vi "calculateGraphData.vi"(7 "Online Buffer (1000)":i32=1000, 8 "error in":errorcluster, 9 "Offset in":i64, 10 "DataBuffers in":dbl[][](array[numeric]), 11 "GraphData in":cluster{dbl[], dbl[]}[](array[cluster])) -> (0 "error out":errorcluster, 3 "GraphData out":cluster{dbl[], dbl[]}[](array[cluster]))   [LabVIEW 2022 SP3, in "StreamReader.lvlib"]
uses:
  <instrlib>/openDAQ/Examples/StreamReader/StreamReader.lvlib
  <vilib>/Utility/miscctls.llb/LVDateTimeRec.ctl
  <vilib>/regexp/Match Regular Expression.xnode
  <instrlib>/openDAQ/Public/Classes/daqUtils/daqUtils.lvlib
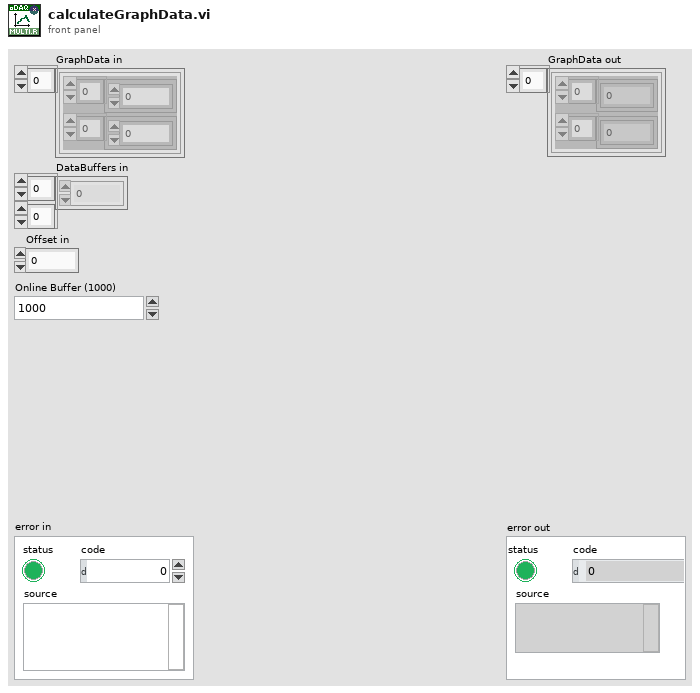
[diagram p1: front panel]
types:
  T1 = enum16{"init", "read", "set sampleRate", "set ruleStart", "set ruleDelta", "set referenceDomainOffset", "set origin", "set unitSymbol", "set resNum", "set resDen", " calculate sampleRate"}
  T2 = typedef "LVDateTimeRec.ctl" = cluster{"fractional second":dbl, "second":i32, "minute":i32, "hour":i32, "day of month":i32, "month":i32, "year":i32, "day of week":i32, "day of year":i32, "DST":i32}
  T3 = typedef "openDAQ.lvlib/DomainMetadata.ctl" = cluster{"sampleRate":i64, "ruleStart":i64, "ruleDelta":i64, "referenceDomainOffset":i64, "origin":string, "unitSymbol":string, "resNum":i64, "resDen":i64}
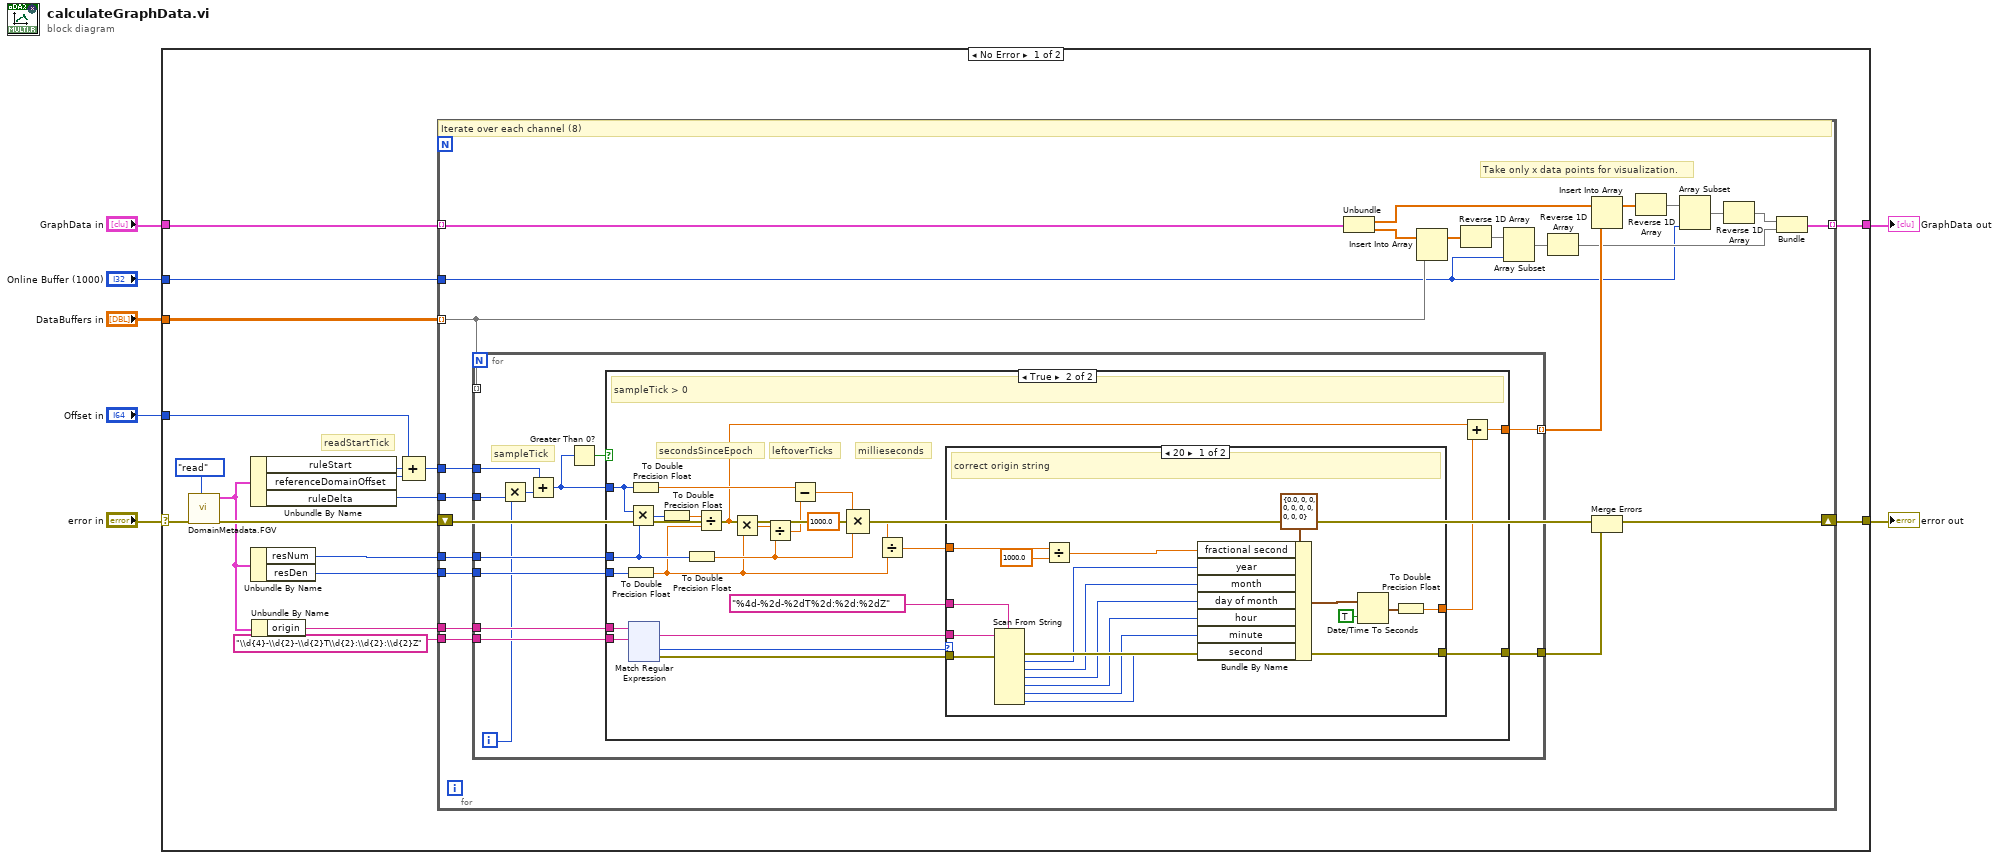
[diagram p0: block diagram]
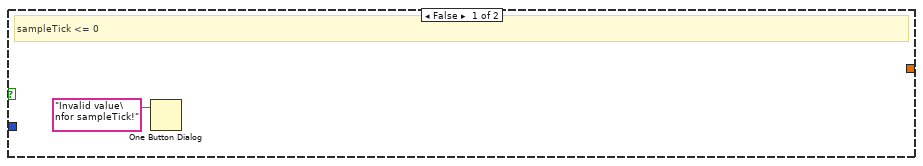
[diagram p2: hidden frame]
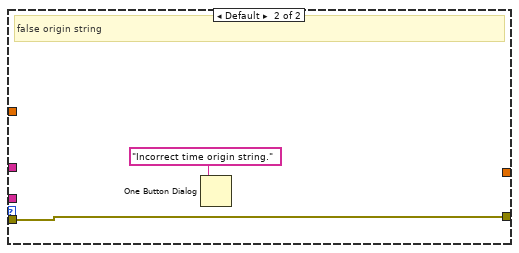
[diagram p3: hidden frame]
diagram:
  n1 = case shown="No Error" "error in" {
    selector: "error in" -> [w9 w225]
    tunnel: [w21 w225] -> w7
    tunnel: "DataBuffers in" -> [w13 _]
    tunnel: "Offset in" -> [w12 _]
    tunnel: "GraphData in" -> [w11 w224]
    tunnel: [w10 w224] -> w3
    tunnel: "Online Buffer (1000)" -> [w8 _]
    frame No Error {
      # "readStartTick"
      n2 = call <instrlib>:"DomainMetadata.FGV.vi"("Case Select"=T1."read", "error in"=w9) -> ("error out"=w22:errorcluster, "DomainMetadata out"=w16:T3)  [unwired: 8 in]
      n3 = Unbundle By Name(w16) -> ("ruleStart"=w24:i64, "referenceDomainOffset"=w23:i64, "ruleDelta"=w19:i64)
      n4 = Unbundle By Name(w16) -> ("resNum"=w18:i64, "resDen"=w17:i64)
      n5 = Unbundle By Name(w16) -> ("origin"=w15:string)
      n6 = Compound Arithmetic op=ADD(w12, w24, w23) -> (w20:i64)
      n7 = for {
        shift-right: [w41] -> w21
        shift-left: w22 -> [w45]
        tunnel: w20 -> [w48]
        tunnel: w19 -> [w49]
        tunnel: w18 -> [w47]
        tunnel: w17 -> [w46]
        tunnel: w15 -> [w44]
        tunnel: "\\d{4}-\\d{2}-\\d{2}T\\d{2}:\\d{2}:\\d{2}Z" ("format string") -> [w43]
        tunnel: w13 -> [w27] mode=indexing
        tunnel: [w39] -> w10 mode=indexing
        tunnel: w11 -> [w38] mode=indexing
        tunnel: w8 -> [w26]
        # "Take only x data points for visualization."
        # "Iterate over each channel (8)"
        n8 = for {
          tunnel: w49 -> [w61]
          tunnel: w48 -> [w59]
          tunnel: w47 -> [w57]
          tunnel: w46 -> [w56]
          tunnel: w44 -> [w54]
          tunnel: w43 -> [w53]
          tunnel: [w52] -> w42
          tunnel: w27 -> [_] mode=indexing
          tunnel: [w50] -> w40 mode=indexing
          i -> [w51]
          # "sampleTick"
          n9 = Multiply(x=w51, y=w61) -> (x*y=w60:i64)
          n10 = Add(x=w59, y=w60) -> (x+y=w55:i64)
          n11 = Greater Than 0?(x=w55) -> (x > 0?=w58:bool)
          n12 = case shown="True" w58 {
            tunnel: w57 -> [_ w82]
            tunnel: w56 -> [_ w84]
            tunnel: w55 -> [_ w81]
            tunnel: w54 -> [_ w69]
            tunnel: w53 -> [_ w73]
            tunnel: [_ w70] -> w52
            tunnel: [_ w63] -> w50
            frame False {
              # "sampleTick <= 0"
              n13 = One Button Dialog(message="Invalid value\nfor sampleTick!") -> ()  [unwired: 1 in, 1 out]
            }
            frame True {
              # "millieseconds"
              # "leftoverTicks"
              # "secondsSinceEpoch"
              # "sampleTick > 0"
              n14 = To Double Precision Float(number=w84) -> (double precision float=w74:dbl)
              n15 = Multiply(x=w81, y=w82) -> (x*y=w86:i64)
              n16 = xnode "Match Regular Expression"("input string"=w69, "regular expression"=w73) -> ("whole match"=w71:string, "offset past match"=w68:i32, "error out"=w67:errorcluster)  [unwired: 4 in, 2 out]
              n17 = To Double Precision Float(number=w81) -> (double precision float=w79:dbl)
              n18 = To Double Precision Float(number=w86) -> (double precision float=w85:dbl)
              n19 = To Double Precision Float(number=w82) -> (double precision float=w76:dbl)
              n20 = Divide(x=w85, y=w74) -> (x/y=w65:dbl)
              n21 = Multiply(x=w65, y=w74) -> (x*y=w83:dbl)
              n22 = Divide(x=w83, y=w76) -> (x/y=w80:dbl)
              n23 = Subtract(x=w79, y=w80) -> (x-y=w78:dbl)
              n24 = Compound Arithmetic op=MULTIPLY(w78, 1000.0 ("x/y"), w76) -> (w75:dbl)
              n25 = Divide(x=w75, y=w74) -> (x/y=w66:dbl)
              n26 = case shown="20" w68 {
                tunnel: "%4d-%2d-%2dT%2d:%2d:%2dZ" ("format string") -> [w220 _]
                tunnel: w71 -> [w219 _]
                tunnel: [w221 w222] -> w70
                tunnel: w67 -> [w218 w222]
                tunnel: [w208 _] -> w64
                tunnel: w66 -> [w206 _]
                frame 20 {
                  # "correct origin string"
                  n27 = Scan From String(format string=w220, input string=w219, error in=w218) -> (error out=w221:errorcluster, output 1=w216:i32, output 2=w215:i32, output 3=w214:i32, output 4=w213:i32, output 5=w212:i32, output 6=w211:i32)  [unwired: 7 in, 2 out]
                  n28 = Divide(x=w206, y=1000.0) -> (x/y=w204:dbl)
                  n29 = Bundle By Name(cluster=T2 {"fractional second"=0.0, "second"=0, "minute"=0, "hour"=0, "day of month"=0, "month"=0, "year"=0, "day of week"=0, "day of year"=0, "DST"=0} ("date time rec"), "fractional second"=w204, "year"=w216, "month"=w215, "day of month"=w214, "hour"=w213, "minute"=w212, "second"=w211) -> (w210:T2)
                  n30 = Date/Time To Seconds(1:TRUE ("is UTC (F)"), 2:w210) -> (0:w209:timestamp)
                  n31 = To Double Precision Float(number=w209) -> (double precision float=w208:dbl)
                }
                frame Default {
                  # "false origin string"
                  n32 = One Button Dialog(message="Incorrect time origin string." ("format string")) -> ()  [unwired: 1 in, 1 out]
                }
              }
              n33 = Add(x=w65, y=w64) -> (x+y=w63:dbl)
            }
          }
        }
        n34 = Unbundle(w38) -> (w37:dbl[], w36:dbl[])
        n35 = Insert Into Array(array=w36, new element=w27) -> (w35:dbl[])  [unwired: 1 in]
        n36 = Reverse 1D Array(array=w35) -> (reversed array=w31:dbl[])
        n37 = Array Subset(array=w31, length=w26) -> (w34:dbl[])  [unwired: 1 in]
        n38 = Reverse 1D Array(array=w34) -> (reversed array=w30:dbl[])
        n39 = Insert Into Array(array=w37, new element=w40) -> (w33:dbl[])  [unwired: 1 in]
        n40 = Merge Errors(w45, w42) -> (w41:errorcluster)
        n41 = Reverse 1D Array(array=w33) -> (reversed array=w29:dbl[])
        n42 = Array Subset(array=w29, length=w26) -> (w32:dbl[])  [unwired: 1 in]
        n43 = Reverse 1D Array(array=w32) -> (reversed array=w28:dbl[])
        n44 = Bundle(w28, w30) -> (w39:cluster{dbl[], dbl[]})  [unwired: 1 in]
      }
    }
    frame Error {
    }
  }
  "error out" <- w7
  "GraphData out" <- w3
